vi "Run Selected Tests.vi"(8 "error in (no error)":errorcluster, 10 "Tests":string[](array[string]), 11 "Execution UI In":refnum<class "Execution UI V2.lvclass">) -> (0 "error out":errorcluster, 3 "Execution UI Out":refnum<class "Execution UI V2.lvclass">)   [LabVIEW 2020, in "Execution UI V2.lvclass"]
uses:
  Execution UI V2.lvclass
  C:/Git/astemes-lunit/source/Rewrite Project/Result Observer/Result Observer.lvclass
  TypeDefs/Execution State.ctl
  Execution UI V2.lvclass/Execution UI V2.ctl
  Test Runner/Test Runner V2.lvclass
  Run/Runnable.lvclass
  Result Model/Result Model.lvclass
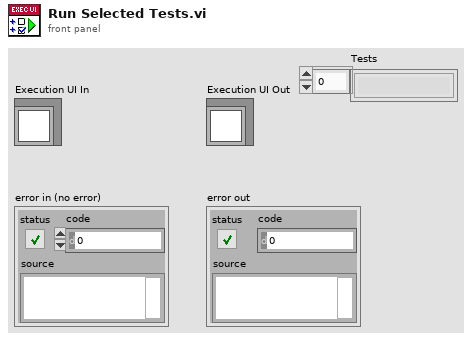
[diagram p1: front panel]
types:
  T1 = typedef "Execution UI V2.lvclass/Execution State.ctl" = enum16{"Idle", "Running"}
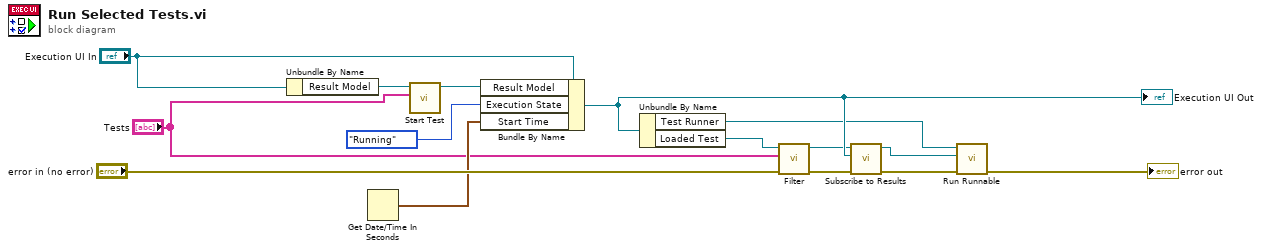
[diagram p0: block diagram]
diagram:
  n1 = Unbundle By Name("Execution UI In") -> ("Result Model"=w14:refnum<class "Result Model.lvclass">)
  n2 = Get Date/Time In Seconds() -> (seconds since 1Jan1904=w2:timestamp)
  n3 = call "Start Test.vi"("Tests"="Tests", "Result Model In"=w14) -> ("Result Model Out"=w13:refnum<class "Result Model.lvclass">)  [unwired: 9 in]
  n4 = Bundle By Name(cluster="Execution UI In", "Result Model"=w13, "Execution State"=Execution_State."Running", "Start Time"=w2) -> (w10:refnum<class "Execution UI V2.lvclass">)
  "Execution UI Out" <- w10
  n5 = Unbundle By Name(w10) -> ("Test Runner"=w3:refnum<class "Test Runner V2.lvclass">, "Loaded Test"=w7:refnum<class "Runnable.lvclass">)
  n6 = call-dynamic "Filter.vi"("error in (no error)"="error in (no error)", "Selected Runnables"="Tests", "Runnable In"=w7) -> ("error out"=w4:errorcluster, "Runnable Out"=w6:refnum<class "Runnable.lvclass">)  [unwired: 7 in]
  n7 = call-dynamic "Subscribe to Results.vi"("error in (no error)"=w4, "Result Observer"=w10, "Runnable In"=w6) -> ("error out"=w8:errorcluster, "Runnable Out"=w9:refnum<class "Runnable.lvclass">)  [unwired: 7 in]
  n8 = call-dynamic "Run Runnable.vi"("error in (no error)"=w8, "Runnable"=w9, "Test Runner"=w3) -> ("error out"=→"error out":errorcluster)  [unwired: 8 in]
